vi "visa_separate_data.vi"(11 "Input string":string) -> (0 "Time":dbl, 1 "Gyro_z":dbl, 2 "Gyro_y":dbl, 3 "Gyro_x":dbl)   [LabVIEW 2019]
panel:
  out "Acc_x":dbl
  out "Acc_y":dbl
  out "Acc_z":dbl
  out "Yaw":dbl
  out "Pitch":dbl
  out "Roll":dbl
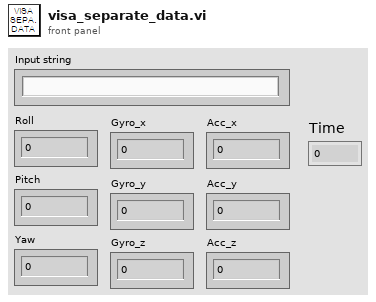
[diagram p1: front panel]
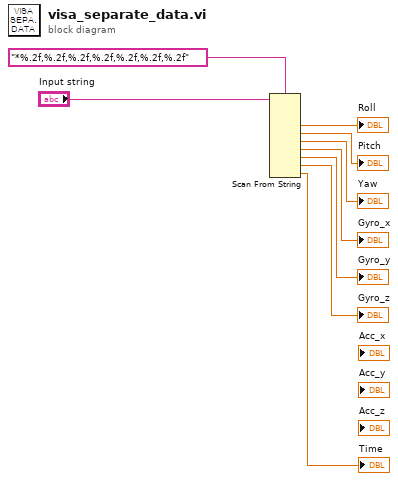
[diagram p0: block diagram]
diagram:
  n1 = Scan From String(format string="*%.2f,%.2f,%.2f,%.2f,%.2f,%.2f,%.2f", input string="Input string") -> (output 1=→"Roll":dbl, output 2=→"Pitch":dbl, output 3=→"Yaw":dbl, output 4=→"Gyro_x":dbl, output 5=→"Gyro_y":dbl, output 6=→"Gyro_z":dbl, output 7=→"Time":dbl)  [unwired: 9 in, 3 out]
